vi "microFPGA_analog_input_addr_60_ctrl.vi"(0 "VISA resource name":refnum<visa-resource-name>, 1 "analog readout channel":u16(ring)=3 items=["channel No 0", "channel No 1", "channel No 2", "channel No 3", "channel No 4", "channel No 5", "channel No 6", "channel No 7", "channel No 8"], 11 "error in (no error)":errorcluster) -> (4 "VISA resource name 2":refnum<visa-resource-name>, 6 "analog value read":i32, 10 "abort_wrong_input":bool, 15 "error out":errorcluster)   [LabVIEW 2018]
panel:
  out "mode read string answer":string
  out "mode read string":string
  out "mode write string":string
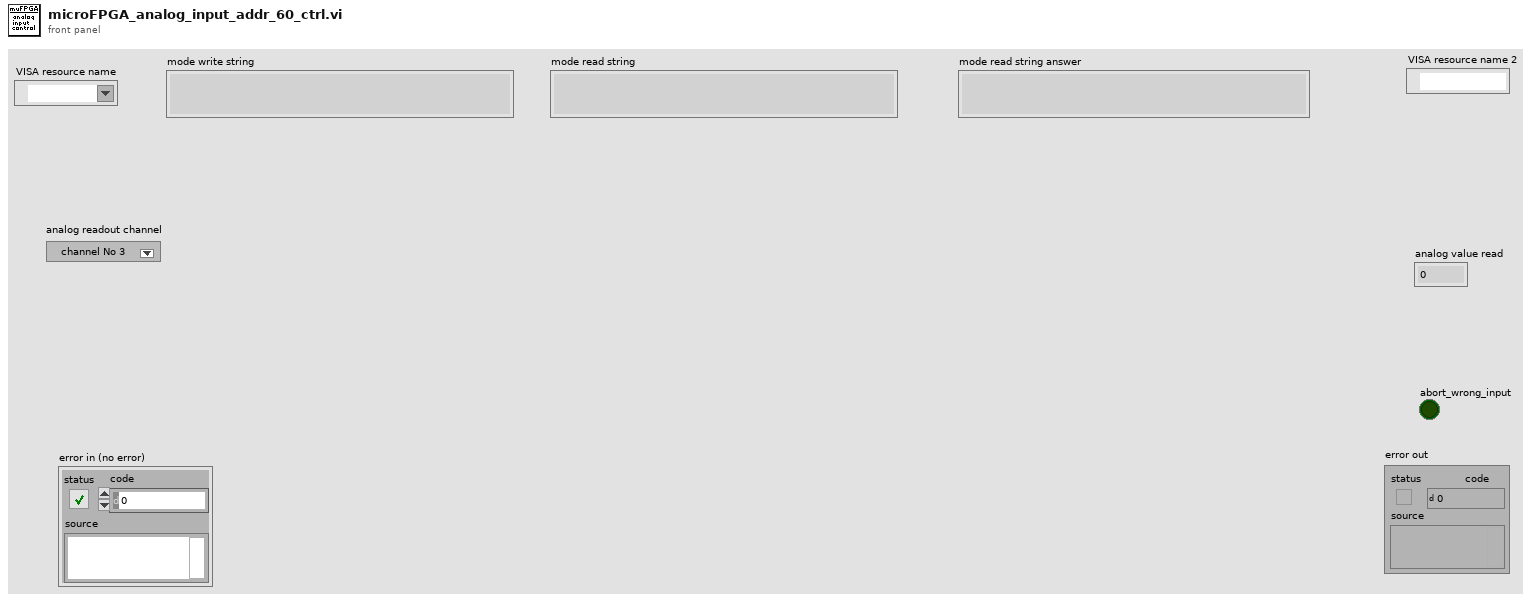
[diagram p1: front panel]
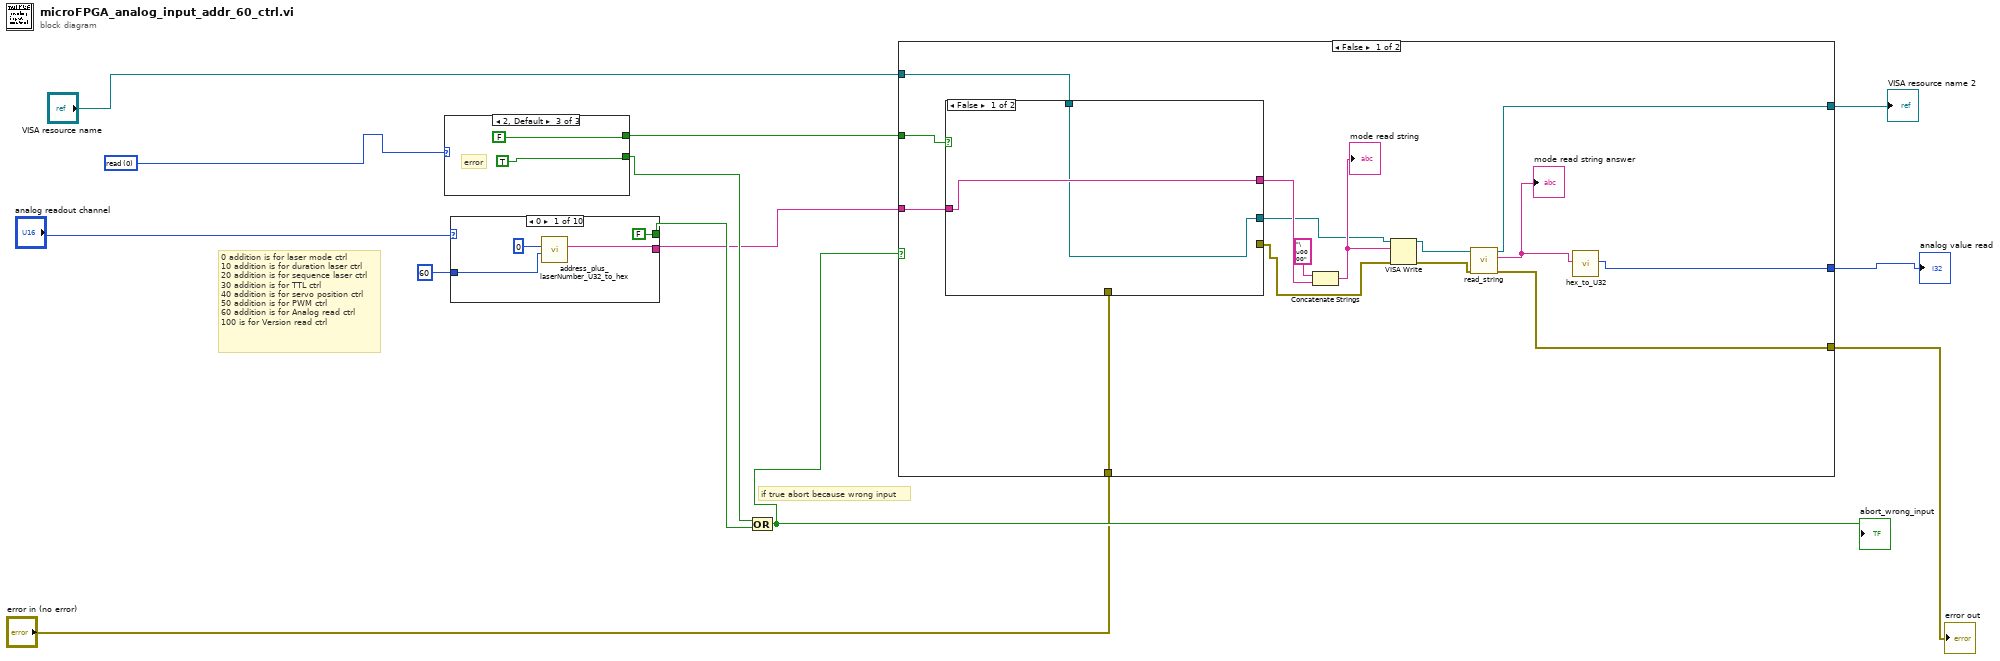
[diagram p0: block diagram]
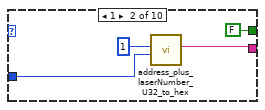
[diagram p2: hidden frame]
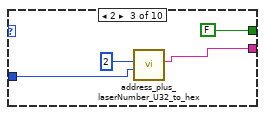
[diagram p3: hidden frame]
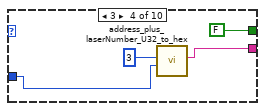
[diagram p4: hidden frame]
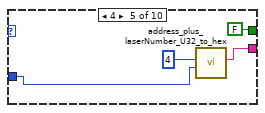
[diagram p5: hidden frame]
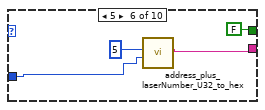
[diagram p6: hidden frame]
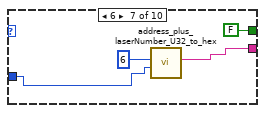
[diagram p7: hidden frame]
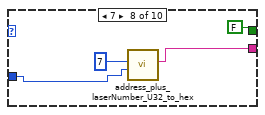
[diagram p8: hidden frame]
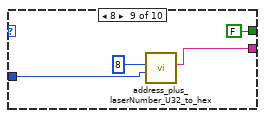
[diagram p9: hidden frame]
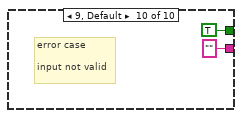
[diagram p10: hidden frame]
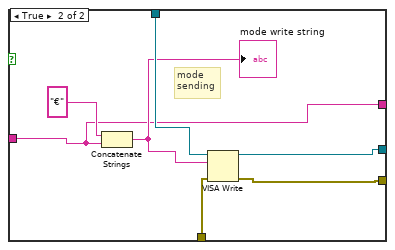
[diagram p11: hidden frame]
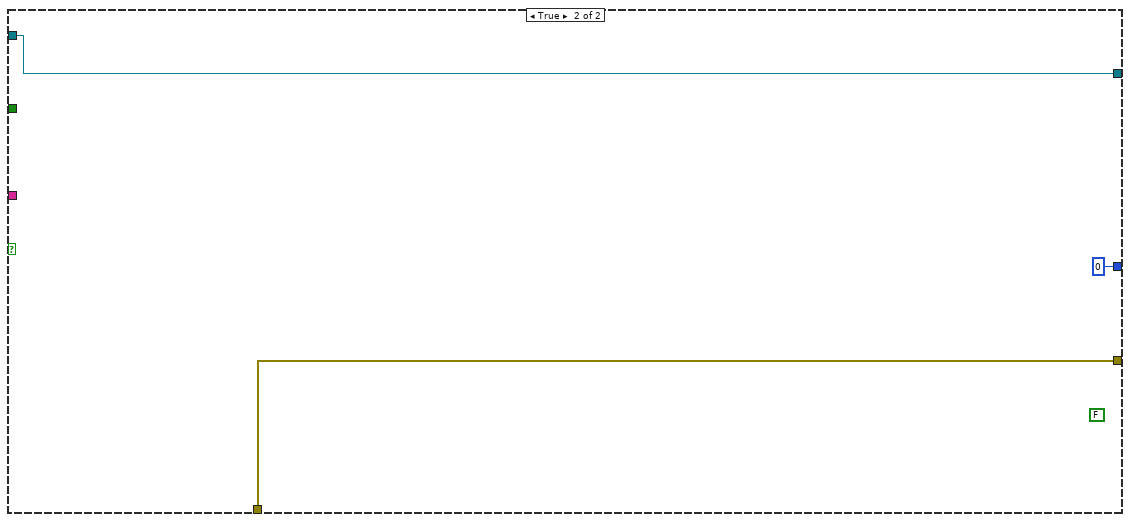
[diagram p12: hidden frame]
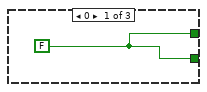
[diagram p13: hidden frame]
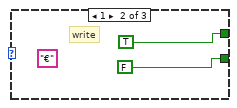
[diagram p14: hidden frame]
diagram:
  w12 = u16 0 items=["read", "write"] ("write or read")
  # "0 addition is for laser mode ctrl\n10 addition is for duration laser ctrl\n20 addition is for sequence laser ctrl\n30 addition is for TTL ctrl\n40 addition is for servo position ctrl\n50 addition is for PWM ctrl\n60 addition is for Analog read ctrl\n100 is for Version read ctrl"
  # "if true abort because wrong input"
  n1 = case shown="2, Default" w12 {
    tunnel: [w14 TRUE FALSE] -> w11
    tunnel: [w14 FALSE TRUE] -> w10
    frame 0 {
      w14 = FALSE
    }
    frame 1 {
      (unwired) "€" ("hex")
      # "write"
    }
    frame 2, Default {
      # "error"
    }
  }
  n2 = case shown="0" "analog readout channel" {
    tunnel: [w20 w24 w28 w32 w36 w40 w44 w47 w53 "" ("string 5")] -> w2
    tunnel: [FALSE FALSE FALSE FALSE FALSE FALSE FALSE FALSE FALSE TRUE] -> w3
    tunnel: u32 60 ("adress offset") -> [w19 w23 w27 w31 w35 w39 w43 w48 w52 _]
    frame 0 {
      n3 = call "address_plus_laserNumber_U32_to_hex.vi"("adress offset"=w19, "y 3"=u32 0) -> ("string 5"=w20:string)  [unwired: 8 in]
    }
    frame 1 {
      n4 = call "address_plus_laserNumber_U32_to_hex.vi"("adress offset"=w23, "y 3"=u32 1) -> ("string 5"=w24:string)  [unwired: 8 in]
    }
    frame 2 {
      n5 = call "address_plus_laserNumber_U32_to_hex.vi"("adress offset"=w27, "y 3"=u32 2) -> ("string 5"=w28:string)  [unwired: 8 in]
    }
    frame 3 {
      n6 = call "address_plus_laserNumber_U32_to_hex.vi"("adress offset"=w31, "y 3"=u32 3) -> ("string 5"=w32:string)  [unwired: 8 in]
    }
    frame 4 {
      n7 = call "address_plus_laserNumber_U32_to_hex.vi"("adress offset"=w35, "y 3"=u32 4) -> ("string 5"=w36:string)  [unwired: 8 in]
    }
    frame 5 {
      n8 = call "address_plus_laserNumber_U32_to_hex.vi"("adress offset"=w39, "y 3"=u32 5) -> ("string 5"=w40:string)  [unwired: 8 in]
    }
    frame 6 {
      n9 = call "address_plus_laserNumber_U32_to_hex.vi"("adress offset"=w43, "y 3"=u32 6) -> ("string 5"=w44:string)  [unwired: 8 in]
    }
    frame 7 {
      n10 = call "address_plus_laserNumber_U32_to_hex.vi"("adress offset"=w48, "y 3"=u32 7) -> ("string 5"=w47:string)  [unwired: 8 in]
    }
    frame 8 {
      n11 = call "address_plus_laserNumber_U32_to_hex.vi"("adress offset"=w52, "y 3"=u32 8) -> ("string 5"=w53:string)  [unwired: 8 in]
    }
    frame 9, Default {
      # "error case\n\ninput not valid"
    }
  }
  n12 = Compound Arithmetic op=OR(w10, w3) -> (w9:bool)
  "abort_wrong_input" <- w9
  n13 = case shown="False" w9 {
    tunnel: "VISA resource name" -> [w71 w82]
    tunnel: w2 -> [w68 _]
    tunnel: w11 -> [w62 _]
    tunnel: [w60 u32 0 ("U32")] -> w1
    tunnel: [w59 w82] -> w8
    tunnel: "error in (no error)" -> [w58 w81]
    tunnel: [w57 w81] -> w6
    frame False {
      n14 = case shown="False" w62 {
        tunnel: w68 -> [w73 w77]
        tunnel: w71 -> [w72 w79]
        tunnel: [w73 w77] -> w69
        tunnel: [w72 w76] -> w64
        tunnel: [_ w75] -> w63
        tunnel: w58 -> [_ w74]
        frame False {
        }
        frame True {
          # "mode \nsending"
          n15 = Concatenate Strings("€" ("string"), w77) -> (w78:string)
          "mode write string" <- w78
          n16 = VISA Write(VISA resource name=w79, write buffer=w78, error in (no error)=w74) -> (VISA resource name out=w76:refnum<visa-resource-name>, error out=w75:errorcluster)  [unwired: 1 out]
        }
      }
      n17 = Concatenate Strings("\u0000" ("string"), w69) -> (w67:string)
      "mode read string" <- w67
      n18 = VISA Write(VISA resource name=w64, write buffer=w67, error in (no error)=w63) -> (VISA resource name out=w66:refnum<visa-resource-name>, error out=w65:errorcluster)  [unwired: 1 out]
      n19 = call "read_string.vi"("error in (no error)"=w65, "VISA resource name 2"=w66) -> ("error out"=w57:errorcluster, "read buffer"=w61:string, "VISA resource name"=w59:refnum<visa-resource-name>)  [unwired: 7 in]
      "mode read string answer" <- w61
      n20 = call "hex_to_U32.vi"("hex"=w61) -> ("U32"=w60:u32)  [unwired: 9 in]
    }
    frame True {
      (unwired) FALSE
    }
  }
  "VISA resource name 2" <- w8
  "error out" <- w6
  "analog value read" <- w1
